vi "SL_Ask Login.vi"() -> (2 "AppKey out":string caption="API Key", 3 "OK?":bool caption="OK")   [LabVIEW 2019]
uses:
  <vilib>/Platform/browser.llb/Open URL in Default Browser (string).vi
panel:
  out "URL out":string caption="URL"
  in  "Help":bool caption="Cancel"
  in  "Cancel":bool
  in  "OK":bool caption="OK2"
  in  "AppKey":string
  in  "URL":string caption="Base URL"
  # "Please enter your SystemLink credentials"
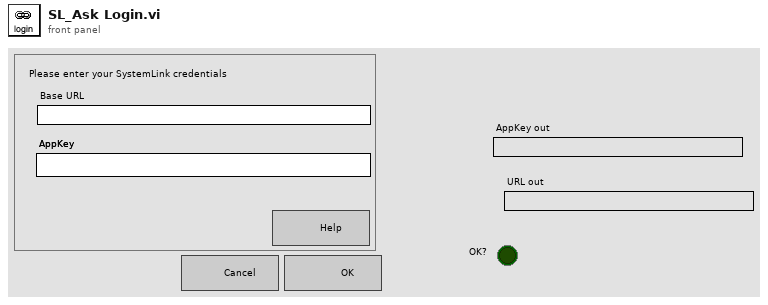
[diagram p1: front panel]
types:
  T1 = enum8{"Enabled", "Disabled", "Disabled and Grayed Out"}
  T2 = cluster{"Name":string, "BaseURL":string, "AppKey":string, "Headers":string[], "Timeout":i32}
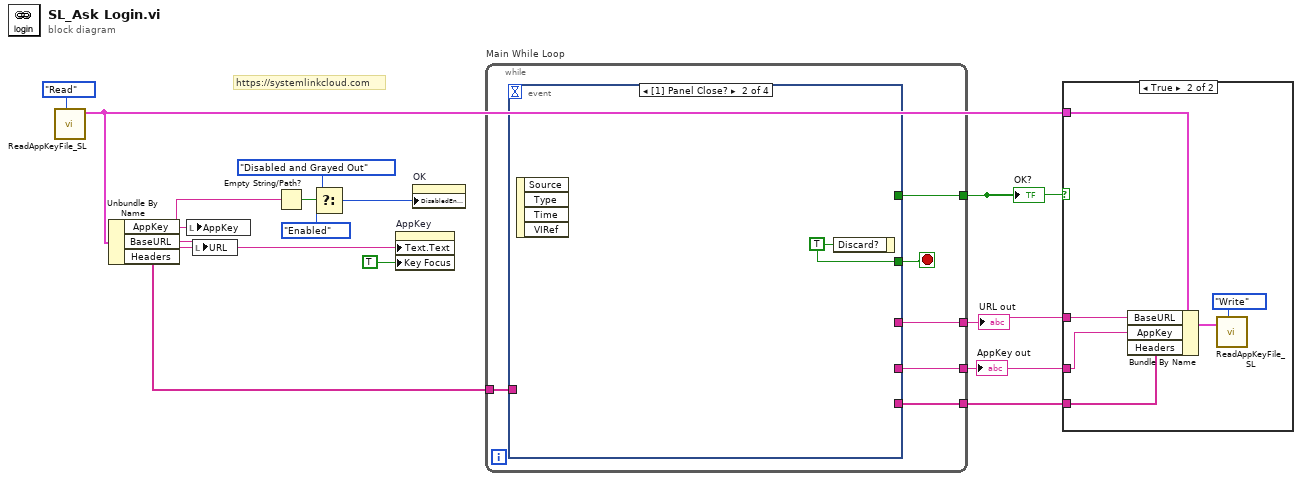
[diagram p0: block diagram]
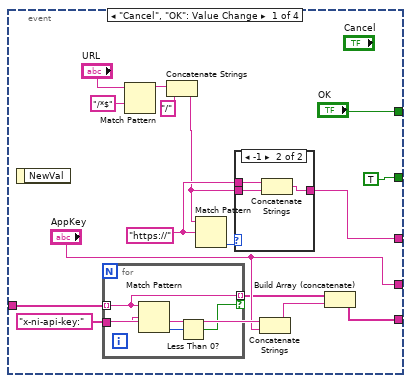
[diagram p3: hidden frame]
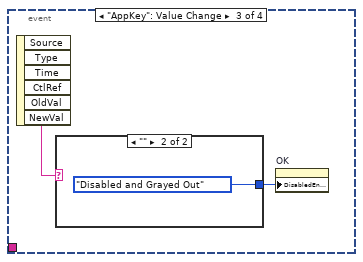
[diagram p5: hidden frame]
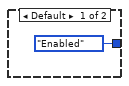
[diagram p6: hidden frame]
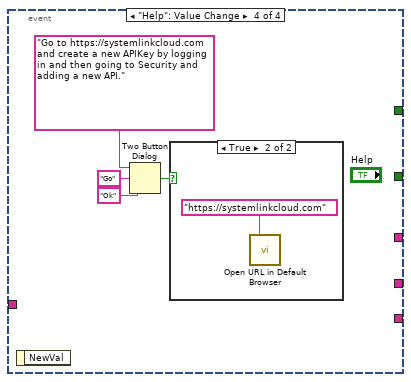
[diagram p7: hidden frame]
diagram:
  # "https://systemlinkcloud.com"
  n1 = call "ReadAppKeyFile_SL.vi"("Task"=enum16{"Read", "Write"}."Read") -> ("Device Out"=w5:T2)  [unwired: 8 in, 2 out]
  n2 = Unbundle By Name(w5) -> ("AppKey"=w8:string, "BaseURL"=w7:string, "Headers"=w2:string[])
  n3 = local write "AppKey"(w8) -> ()
  n4 = local write "URL"(w7) -> ()
  n5 = Empty String/Path?(string/path=w8) -> (empty?=w12:bool)
  n6 = Select(t=T1."Disabled and Grayed Out" ("Disabled"), s=w12, f=T1."Enabled" ("Disabled")) -> (s? t:f=w9:T1)
  n7 = property on="AppKey" class="Str"("Text.Text"=w8, "Key Focus"=TRUE ("focus on")) -> ()  [unwired: 2 in, 2 out]
  n8 = property on="OK" class="Bool"("DisabledEnum"=w9) -> ()  [unwired: 2 in, 2 out]
  n9 = while "Main While Loop" {
    tunnel: [w19] -> w6
    tunnel: [w18] -> w4
    tunnel: [w17] -> w3
    tunnel: w2 -> [w16]
    tunnel: [w15] -> w1
    stop <- w20 stop-if-true
    n10 = event shown="[1] Panel Close?" {
      selector: _ -> [_ _ _ _]
      dyn-events: _ -> [_ _ _ _]
      timeout: _ -> [_ _ _ _]
      tunnel: [TRUE w45 _ _] -> w20
      tunnel: ["OK" _ _ _] -> w19
      tunnel: [w32 _ _ _] -> w18
      tunnel: ["AppKey" _ _ _] -> w17
      tunnel: [w26 _ _ _] -> w15
      tunnel: w16 -> [w31 _ _ _]
      event "Cancel", "OK": Value Change {
        w30 = "x-ni-api-key:" ("regular expression")
        w33 = "https://" ("URL")
        n11 = event-data() -> ()  [unwired: 1 in, 1 out]
        n12 = for {
          tunnel: w31 -> [w40] mode=indexing
          tunnel: [w40] -> w28 mode=indexing if=w38
          tunnel: w30 -> [w37]
          n13 = Match Pattern(string=w40, regular expression=w37) -> (offset past match=w39:i32)  [unwired: 1 in, 3 out]
          n14 = Less Than 0?(x=w39) -> (x < 0?=w38:bool)
        }
        n15 = Match Pattern(string="URL", regular expression="/*$") -> (before substring=w23:string)  [unwired: 1 in, 3 out]
        n16 = Concatenate Strings(w23, "/" ("regular expression")) -> (w21:string)
        n17 = Match Pattern(string=w21, regular expression=w33) -> (offset past match=w34:i32)  [unwired: 1 in, 3 out]
        n18 = case shown="-1" w34 {
          tunnel: w33 -> [_ w44]
          tunnel: w21 -> [w41 w43]
          tunnel: [w41 w42] -> w32
          frame Default {
          }
          frame -1 {
            n19 = Concatenate Strings(w44, w43) -> (w42:string)
          }
        }
        n20 = Concatenate Strings(w30, "AppKey") -> (w27:string)
        n21 = Build Array (concatenate)(w28, w27) -> (w26:string[])
      }
      event Panel Close? {
        w45 = TRUE ("Discard?")
        n22 = event-data() -> ()  [unwired: 1 in, 4 out]
        n23 = event-data("Discard?"=w45) -> ()  [unwired: 1 in, 1 out]
      }
      event "AppKey": Value Change {
        n24 = event-data() -> ("NewVal"=w46:string)  [unwired: 1 in, 5 out]
        n25 = case shown="\"\"" w46 {
          tunnel: [T1."Enabled" ("Disabled") T1."Disabled and Grayed Out" ("Disabled")] -> w47
          frame Default {
          }
          frame "" {
          }
        }
        n26 = property on="OK" class="Bool"("DisabledEnum"=w47) -> ()  [unwired: 2 in, 2 out]
      }
      event "Help": Value Change {
        n27 = event-data() -> ()  [unwired: 1 in, 1 out]
        n28 = Two Button Dialog(message="Go to https://systemlinkcloud.com and create a new APIKey by logging in and then going to Security and adding a new API.", 1:"Ok" ("F button name (\"Cancel\")"), 2:"Go" ("T button name (\"OK\")")) -> (T button?=w50:bool)
        n29 = case shown="True" w50 {
          frame False {
          }
          frame True {
            n30 = call-poly <vilib>:"Open URL in Default Browser.vi"("URL"="https://systemlinkcloud.com" ("T button name (\"OK\")")) -> ()  [unwired: 5 in, 2 out]
          }
        }
      }
    }
  }
  "AppKey out" <- w3
  "URL out" <- w4
  "OK?" <- w6
  n31 = case shown="True" w6 {
    tunnel: w5 -> [_ w59]
    tunnel: w4 -> [_ w58]
    tunnel: w3 -> [_ w57]
    tunnel: w1 -> [_ w55]
    frame False {
    }
    frame True {
      n32 = Bundle By Name(cluster=w59, "BaseURL"=w58, "AppKey"=w57, "Headers"=w55) -> (w56:T2)
      n33 = call "ReadAppKeyFile_SL.vi"("Task"=enum16{"Read", "Write"}."Write", "Device In"=w56) -> ()  [unwired: 7 in, 3 out]
    }
  }
